vi "myRIOCompareDeviceFamily.vi"(8 "Last Device Code":string, 11 "Device Code":string) -> (3 "Same family?":bool)   [LabVIEW 2021]
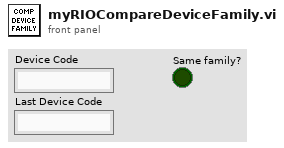
[diagram p1: front panel]
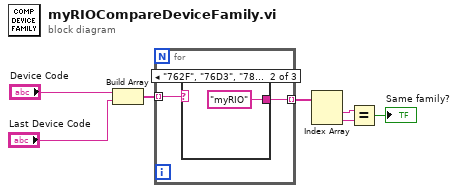
[diagram p0: block diagram]
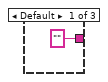
[diagram p2: hidden frame]
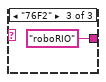
[diagram p3: hidden frame]
diagram:
  n1 = Build Array("Device Code", "Last Device Code") -> (w5:string[])
  n2 = for {
    tunnel: w5 -> [w9] mode=indexing
    tunnel: [w8] -> w4 mode=indexing
    n3 = case shown="\"762F\", \"76D3\", \"7885\"" w9 {
      tunnel: ["" "myRIO" "roboRIO"] -> w8
      frame Default {
      }
      frame "762F", "76D3", "7885" {
      }
      frame "76F2" {
      }
    }
  }
  n4 = Index Array(array=w4) -> (element #1=w3:string, element #2=w2:string)  [unwired: 2 in]
  n5 = Equal?(x=w3, y=w2) -> (x = y?=→"Same family?":bool)
